vi "serverInstancesTest.vi"(8 "error in (no error)":errorcluster) -> (0 "error out":errorcluster)   [LabVIEW 2018]
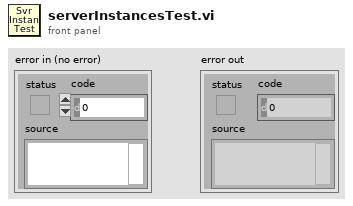
[diagram p1: front panel]
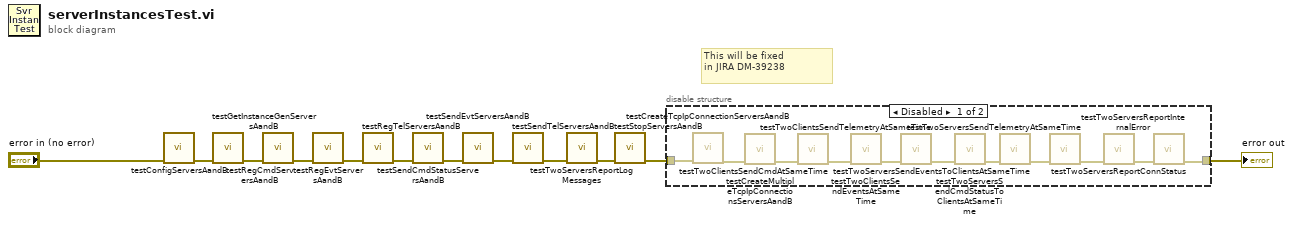
[diagram p0: block diagram]
diagram:
  # "This will be fixed\nin JIRA DM-39238"
  n1 = call "testConfigServersAandB.vi"("error in (no error)"="error in (no error)") -> ("error out"=w3:errorcluster)  [unwired: 10 in]
  n2 = call "testGetInstanceGenServersAandB.vi"("error in (no error)"=w3) -> ("error out"=w2:errorcluster)  [unwired: 10 in]
  n3 = call "testRegCmdServersAandB.vi"("error in (no error)"=w2) -> ("error out"=w8:errorcluster)  [unwired: 10 in]
  n4 = call "testRegEvtServersAandB.vi"("error in (no error)"=w8) -> ("error out"=w7:errorcluster)  [unwired: 10 in]
  n5 = call "testRegTelServersAandB.vi"("error in (no error)"=w7) -> ("error out"=w6:errorcluster)  [unwired: 10 in]
  n6 = call "testSendCmdStatusServersAandB.vi"("error in (no error)"=w6) -> ("error out"=w5:errorcluster)  [unwired: 10 in]
  n7 = call "testSendEvtServersAandB.vi"("error in (no error)"=w5) -> ("error out"=w4:errorcluster)  [unwired: 10 in]
  n8 = call "testSendTelServersAandB.vi"("error in (no error)"=w4) -> ("error out"=w1:errorcluster)  [unwired: 10 in]
  n9 = call "testTwoServersReportLogMessages.vi"("error in"=w1) -> ("error out"=w10:errorcluster)  [unwired: 10 in]
  n10 = call "testStopServersAandB.vi"("error in (no error)"=w10) -> ("error out"=w11:errorcluster)  [unwired: 10 in]
  n11 = disable-structure shown="Disabled" {
    disable-tunnel: w11 -> [w23 w24]
    disable-tunnel: [w13 w24] -> w9
    frame Disabled {
      n12 = call "testCreateTcpIpConnectionServersAandB.vi"("error in"=w23) -> ("error out"=w22:errorcluster)  [unwired: 10 in]
      n13 = call "testCreateMultipleTcpIpConnectionsServersAandB.vi"("error in"=w22) -> ("error out"=w21:errorcluster)  [unwired: 10 in]
      n14 = call "testTwoClientsSendCmdAtSameTime.vi"("error in"=w21) -> ("error out"=w20:errorcluster)  [unwired: 10 in]
      n15 = call "testTwoClientsSendEventsAtSameTime.vi"("error in"=w20) -> ("error out"=w19:errorcluster)  [unwired: 10 in]
      n16 = call "testTwoClientsSendTelemetryAtSameTime.vi"("error in"=w19) -> ("error out"=w18:errorcluster)  [unwired: 10 in]
      n17 = call "testTwoServersSendCmdStatusToClientsAtSameTime.vi"("error in"=w18) -> ("error out"=w17:errorcluster)  [unwired: 10 in]
      n18 = call "testTwoServersSendEventsToClientsAtSameTime.vi"("error in"=w17) -> ("error out"=w16:errorcluster)  [unwired: 10 in]
      n19 = call "testTwoServersSendTelemetryAtSameTime.vi"("error in"=w16) -> ("error out"=w15:errorcluster)  [unwired: 10 in]
      n20 = call "testTwoServersReportConnStatus.vi"("error in"=w15) -> ("error out"=w14:errorcluster)  [unwired: 10 in]
      n21 = call "testTwoServersReportInternalError.vi"("error in"=w14) -> ("error out"=w13:errorcluster)  [unwired: 10 in]
    }
    frame Enabled {
    }
  }
  "error out" <- w9
